vi "(SubVI)Launcher_XOR Encryption & Hash.vi"(7 "Hex String? (t)":bool=TRUE, 8 "error in (no error)":errorcluster caption="에러 입력(에러 없음)", 11 "Plain Text":string) -> (0 "error out":errorcluster caption="에러 출력", 2 "XOR Encrypted Hex Str":string, 3 "Digest":string)   [LabVIEW 2020]
uses:
  <vilib>/security/Message Digest/API/Instances/Byte Array/SHA3-256 Byte Array Checksum.vi
  <vilib>/security/Message Digest/API/NI_Message Digest API.lvlib
panel:
  out "GUID":string="7770365D-F84E-4489-90E9-F0D9D9D97EEF"
  out "XOR Encryption Key Hex Str":string
  out "XOR Encryption Key U8":u8[](array[numeric])=[130, 29, 76, 242, 185, 50, 73, 189, 133, 152, 54, 194, 155, 6, 96, 242] format="%02x"
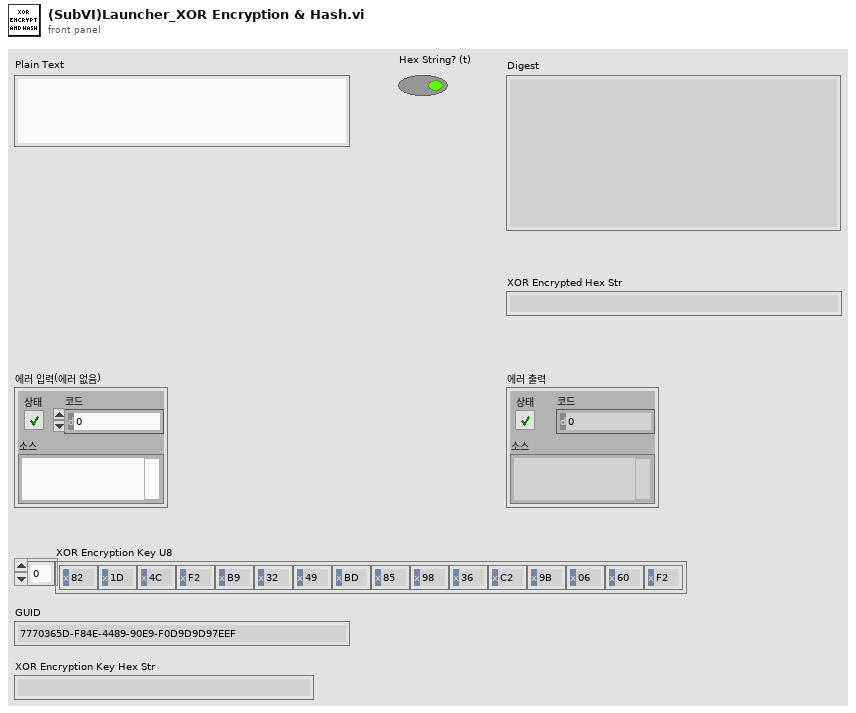
[diagram p1: front panel]
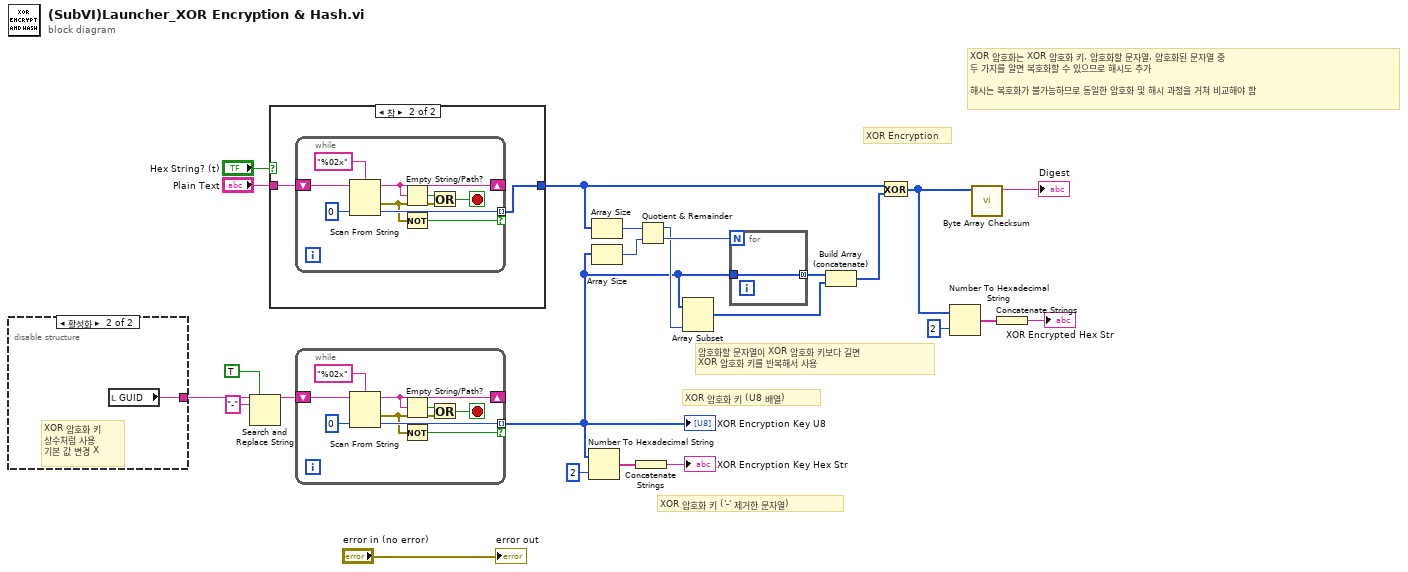
[diagram p0: block diagram]
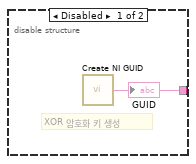
[diagram p2: hidden frame]
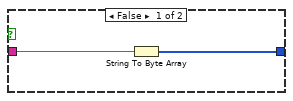
[diagram p3: hidden frame]
diagram:
  # "XOR 암호화는 XOR 암호화 키, 암호화할 문자열, 암호화된 문자열 중\n두 가지를 알면 복호화할 수 있으므로 해시도 추가\n\n해시는 복호화가 불가능하므로 동일한 암호화 및 해시 과정을 거쳐 비교해야 함"
  # "암호화할 문자열이 XOR 암호화 키보다 길면\nXOR 암호화 키를 반복해서 사용"
  # "XOR 암호화 키 ('-' 제거한 문자열)"
  # "XOR 암호화 키 (U8 배열)"
  # "XOR Encryption"
  n1 = disable-structure shown="활성화" {
    disable-tunnel: [w25 w26] -> w2
    frame Disabled {
      # "XOR 암호화 키 생성"
      n2 = call <vilib>:"Create NI GUID.vi"() -> ("NI GUID"=w25:string)
      "GUID" <- w25
    }
    frame Enabled {
      # "XOR 암호화 키\n상수처럼 사용\n기본 값 변경 X"
      n3 = local read "GUID"() -> (w26:string)
    }
  }
  n4 = Search and Replace String(replace all?=TRUE ("모두 대체? (거짓)"), input string=w2, search string="-" ("검색 문자열")) -> (result string=w3:string)  [unwired: 5 in, 3 out]
  n5 = case shown="참" "Hex String? (t)" {
    tunnel: "Plain Text" -> [w28 w30]
    tunnel: [w27 w29] -> w16
    frame False {
      n6 = String To Byte Array(string=w28) -> (unsigned byte array=w27:u8[])
    }
    frame True {
      n7 = while {
        shift-right: [w36] -> _
        shift-left: w30 -> [w39]
        tunnel: [w33] -> w29 mode=indexing if=w31
        stop <- w34 stop-if-true
        n8 = Scan From String(format string="%02x" ("포맷 문자열"), input string=w39, default 1=u8 0) -> (remaining string=w36:string, error out=w32:errorcluster, output 1=w33:u8)  [unwired: 2 in, 1 out]
        n9 = Empty String/Path?(string/path=w36) -> (empty?=w35:bool)
        n10 = Not(x=w32) -> (.not. x?=w31:bool)
        n11 = Or(x=w35, y=w32) -> (x .or. y?=w34:bool)
      }
    }
  }
  n12 = while {
    shift-right: [w45] -> _
    shift-left: w3 -> [w48]
    tunnel: [w42] -> w7 mode=indexing if=w40
    stop <- w43 stop-if-true
    n13 = Scan From String(format string="%02x" ("포맷 문자열"), input string=w48, default 1=u8 0) -> (remaining string=w45:string, error out=w41:errorcluster, output 1=w42:u8)  [unwired: 2 in, 1 out]
    n14 = Empty String/Path?(string/path=w45) -> (empty?=w44:bool)
    n15 = Not(x=w41) -> (.not. x?=w40:bool)
    n16 = Or(x=w44, y=w41) -> (x .or. y?=w43:bool)
  }
  "XOR Encryption Key U8" <- w7
  n17 = Number To Hexadecimal String(1:i16 2 ("폭(-)"), 2:w7) -> (0:w8:string[])
  n18 = Array Size(array=w16) -> (size(s)=w22:i32)
  n19 = Array Size(array=w7) -> (size(s)=w21:i32)
  n20 = Concatenate Strings(w8) -> (→"XOR Encryption Key Hex Str":string)
  n21 = Quotient & Remainder(x=w22, y=w21) -> (x-y*floor(x/y)=w18:i32, floor(x/y)=w20:i32)
  n22 = Array Subset(array=w7, length=w18) -> (w17:u8[])  [unwired: 1 in]
  n23 = for {
    N: w20 -> [_]
    tunnel: w7 -> [w49]
    tunnel: [w49] -> w19 mode=concatenating
  }
  n24 = Build Array (concatenate)(w19, w17) -> (w15:u8[])
  n25 = Exclusive Or(1:w15, 2:w16) -> (0:w14:u8[])
  n26 = Number To Hexadecimal String(1:i16 2 ("폭(-)"), 2:w14) -> (0:w13:string[])
  n27 = call-poly <vilib>:"Byte Array Checksum.vi"("buffer"=w14) -> ("digest"=→"Digest":string)  [unwired: 10 in]
  n28 = Concatenate Strings(w13) -> (→"XOR Encrypted Hex Str":string)
  "error out" <- "error in (no error)"
